vi "matlabGenStackScript.vi"(1 "noImgsInStack":dbl=201.0, 2 "tifStackFname":string="C:\\Users\\sims01\\Desktop\\contAcqDataTest\\chan0_yPos0_xPos0.tif", 3 "stackFnameBase":string="C:\\Users\\sims01\\Desktop\\contAcqDataTest\\chan0_yPos0_xPos0") -> (0 "No stacksGenerated":dbl=1.0)   [LabVIEW 2015]
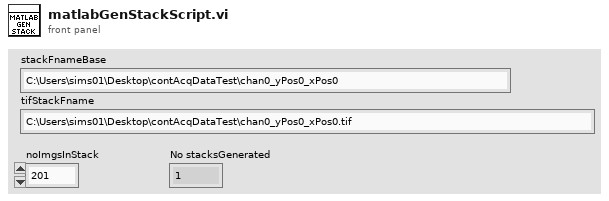
[diagram p1: front panel]
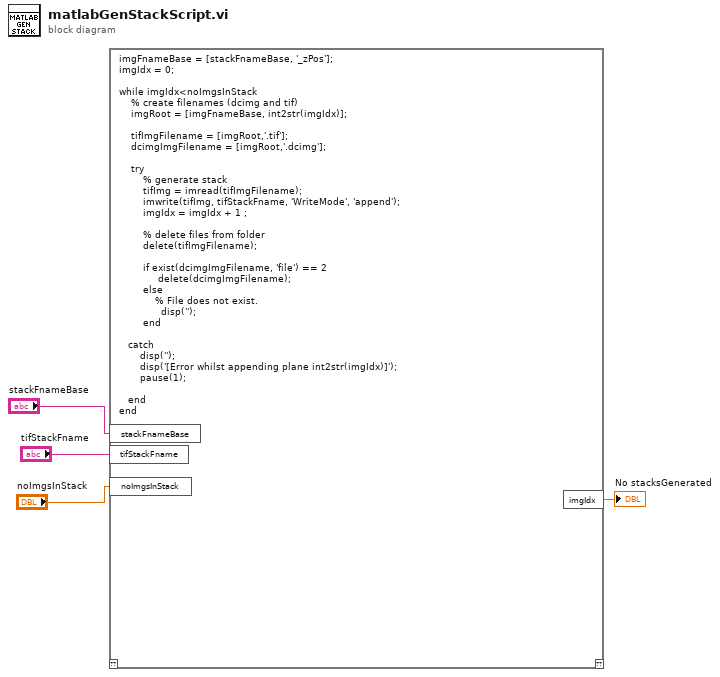
[diagram p0: block diagram]
diagram:
  n1 = script code="imgFnameBase = [stackFnameBase, '_zPos'];\nimgIdx = 0;\n\nwhile imgIdx<noImgsInStack \n    % create filenames (dcimg and tif)\n    imgRoot = [imgFnameBase, int2str(imgIdx)];\n    \n    tifImgFilename = [imgRoot,'.tif'];\n    dcimgImgFilename = [imgRoot,'.dcimg'];\n    \n    try\n        % generate stack\n        tifImg = imread(tifImgFilename);\n        imwrite(tifImg, tifStackFname, 'WriteMode', 'append');\n        imgIdx = imgIdx + 1 ; \n\n        % delete files from folder\n        delete(tifImgFilename);\n        \n        if exist(dcimgImgFilename, 'file') == 2\n             delete(dcimgImgFilename);\n        else\n            % File does not exist.\n              disp('');\n        end\n\n   catch\n       disp('');\n       disp('[Error whilst appending plane int2str(imgIdx)]');\n       pause(1);\n   \n   end\nend"("tifStackFname"="tifStackFname", "stackFnameBase"="stackFnameBase", "noImgsInStack"="noImgsInStack") -> ("imgIdx"=→"No stacksGenerated":dbl)  [unwired: 1 in, 1 out]
